vi "Get All.vi"(0 "Tree Reference In":refnum<vi>, 2 "Starting Tag":string, 3 "Input Tree Items(DO NOT WIRE)":string[](array[string]), 5 "error in (no error)":errorcluster) -> (14 "Tree Reference Out":refnum<vi>, 16 "Current Item":string, 17 "Output Tree Items":string[](array[string]), 19 "error out":errorcluster)   [LabVIEW 2015, in "QuickVIew.lvlib"]
doc: "Retrieves all elements in tree at and below the starting tag. When Starting Tag and Input Tree Items are left unwired it will return all elements in the tree. TLB Prime - Application Template 1.3.0.24\nNorm Kirchner, NI Systems Engineering - NI\nCopyright (c) 2014, NI"
uses:
  QuickVIew.lvlib
panel:
  in  "Identical VI Refnum":refnum<vi>
  # "VI LOCALS"
  # "VI OUTPUTS"
  # "VI INPUTS"
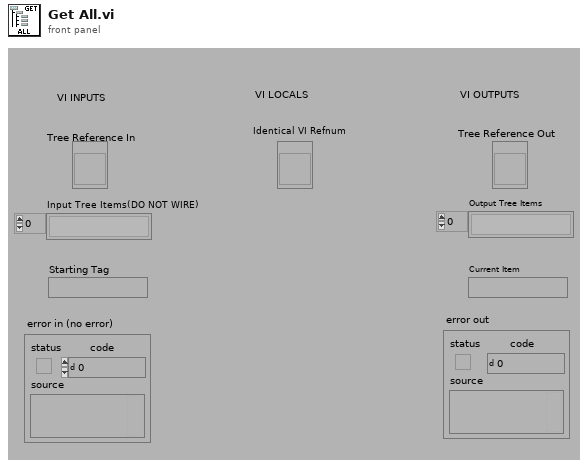
[diagram p1: front panel]
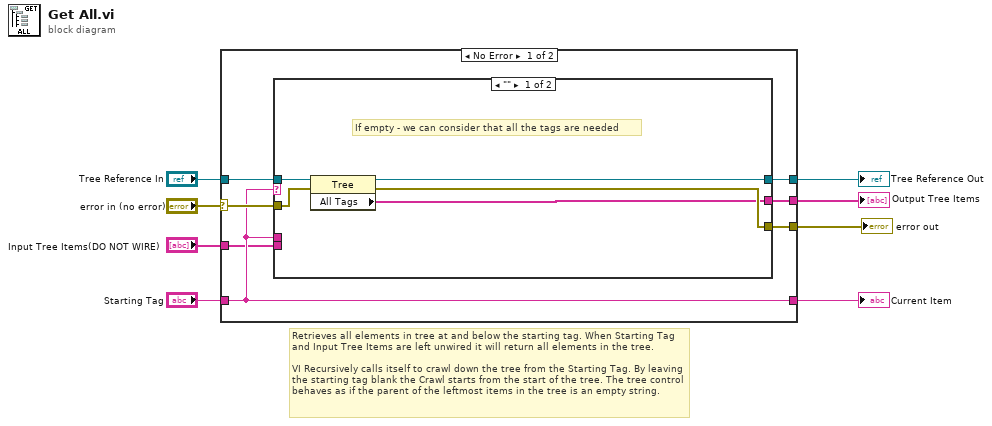
[diagram p0: block diagram]
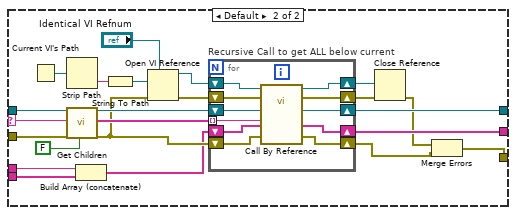
[diagram p2: hidden frame]
diagram:
  # "Retrieves all elements in tree at and below the starting tag. When Starting Tag and Input Tree Items are left unwired it will return all elements in the tree. \n\nVI Recursively calls itself to crawl down the tree from the Starting Tag. By leaving the starting tag blank the Crawl starts from the start of the tree. The tree control behaves as if the parent of the leftmost items in the tree is an empty string."
  n1 = case shown="No Error" "error in (no error)" {
    selector: "error in (no error)" -> [w11 w55]
    tunnel: "Tree Reference In" -> [w15 w56]
    tunnel: [w14 w56] -> w7
    tunnel: "Starting Tag" -> [w10 w58]
    tunnel: [w13 w57] -> w5
    tunnel: [w10 w58] -> w4
    tunnel: "Input Tree Items(DO NOT WIRE)" -> [w9 w57]
    tunnel: [w12 w55] -> w1
    frame No Error {
      n2 = case shown="\"\"" w10 {
        selector: w10 -> [_ w24]
        tunnel: w15 -> [w20 w43]
        tunnel: [w18 w42] -> w14
        tunnel: [w16 w41] -> w13
        tunnel: [w17 w25] -> w12
        tunnel: w11 -> [w19 w29]
        tunnel: w10 -> [_ w23]
        tunnel: w9 -> [_ w22]
        frame "" {
          # "If empty - we can consider that all the tags are needed"
          n3 = property class="Tree"(reference=w20, error in=w19) -> (reference out=w18:refnum<vi>, error out=w17:errorcluster, "All Tags"=w16:string[])
        }
        frame Default {
          n4 = Current VI's Path() -> (path=w34:path)
          n5 = Strip Path(path=w34) -> (name=w32:string)  [unwired: 1 out]
          n6 = call "Get Children.vi"("Tree Reference In"=w43, "Parent Tag"=w24, "error in (no error)"=w29, "Use Current"=FALSE) -> ("Tree Reference Out"=w40:refnum<vi>, "Children Tags"=w36:string[], "error out"=w28:errorcluster)  [unwired: 13 out]
          n7 = Build Array (concatenate)(w23, w22) -> (w21:string[])
          n8 = String To Path(string=w32) -> (path=w33:path)
          n9 = Open VI Reference(type specifier VI Refnum (for type only)="Identical VI Refnum", vi path=w33, error in (no error)=w28) -> (vi reference=w35:refnum<vi>, error out=w38:errorcluster)  [unwired: 1 in, 2 out]
          n10 = for "Recursive Call to get ALL below current" {
            shift-right: [w52] -> w26
            shift-left: w28 -> [w53]
            shift-right: [w51] -> w42
            shift-left: w40 -> [w54]
            shift-right: [w48] -> w37
            shift-left: w38 -> [w49]
            shift-right: [w44] -> w39
            shift-left: w35 -> [w50]
            tunnel: w36 -> [w47] mode=indexing
            shift-right: [w46] -> w41
            shift-left: w21 -> [w45]
            n11 = call-by-ref "?"(reference=w50, error in=w49, "Tree Reference In"=w54, "Starting Tag"=w47, "Input Tree Items(DO NOT WIRE)"=w45, "error in (no error)"=w53) -> (reference out=w44:refnum<vi>, error out=w48:errorcluster, "Tree Reference Out"=w51:refnum<vi>, "Output Tree Items"=w46:string[], 19:"error out"=w52:errorcluster)  [unwired: 12 in, 1 out]
          }
          n12 = Close Reference(reference=w39, error in (no error)=w37) -> (error out=w27:errorcluster)
          n13 = Merge Errors(w27, w26) -> (w25:errorcluster)
        }
      }
    }
    frame Error {
    }
  }
  "error out" <- w1
  "Tree Reference Out" <- w7
  "Output Tree Items" <- w5
  "Current Item" <- w4
